vi "nested for loop.vi"() -> ()   [LabVIEW 2012]
panel:
  out "Array":i32[][](array[numeric])
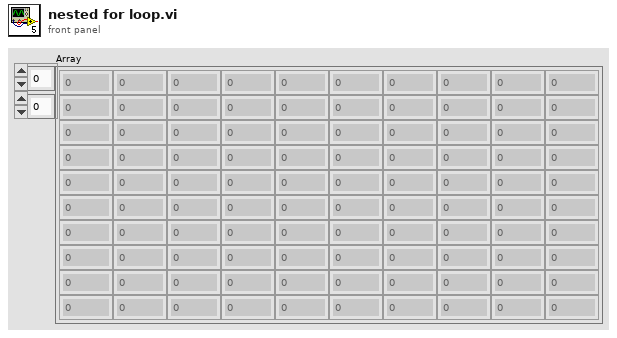
[diagram p1: front panel]
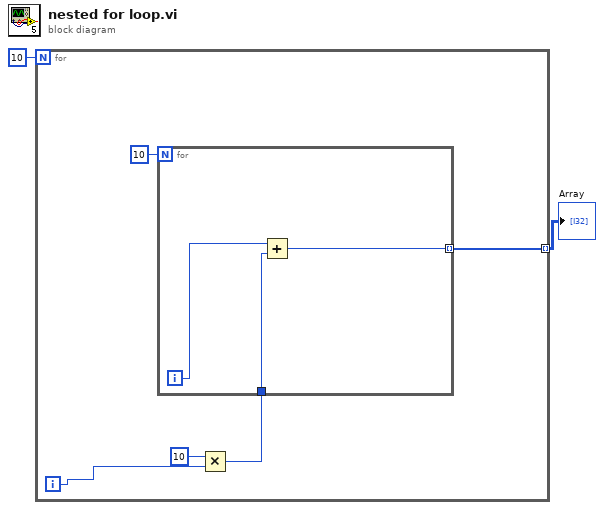
[diagram p0: block diagram]
diagram:
  n1 = for {
    N: 10 -> [_]
    tunnel: [w6] -> w1 mode=indexing
    i -> [w4]
    n2 = Multiply(x=10, y=w4) -> (x*y=w5:i32)
    n3 = for {
      N: 10 -> [_]
      tunnel: [w10] -> w6 mode=indexing
      tunnel: w5 -> [w8]
      i -> [w9]
      n4 = Add(x=w9, y=w8) -> (x+y=w10:i32)
    }
  }
  "Array" <- w1
